vi "Move_Axis_tl.vi"(2 "GOTO":dbl step=1.0 format="%.5f", 3 "Mode":enum16{"Move", "Teach"}(ring), 4 "AXIS":T2 items=["Spare 0", "X", "Y", "Z", "THETA", "PHI", "Spare 6"]) -> (0 "ACTUAL POS.":dbl step=0.00125 format="%.5f", 1 "CURRENT POSITIONS":T1[](array[typedef])=[{"axis"="X", "mac position"=0.0}, {"axis"="Y", "mac position"=0.0}, {"axis"="Z", "mac position"=0.0}, {"axis"="PHI", "mac position"=0.0}, {"axis"="THETA", "mac position"=0.0}] {"mac position" format="%.5f"})   [LabVIEW 2010]
uses:
  TRAVERSE SUB-VIs/Custom Controls/Axis_Control_tl.ctl
  TRAVERSE SUB-VIs/Custom Controls/Axis_pos_cluster_tl.ctl
  TRAVERSE SUB-VIs/Functional VIs/Traverse_setup_tl.glob.vi
panel:
  in  "ADJUST PARAMETERS?":bool=TRUE
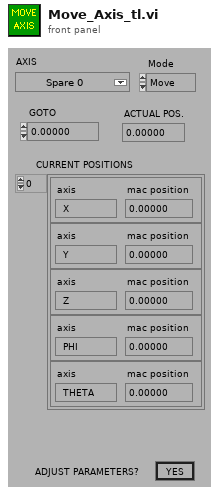
[diagram p1: front panel]
types:
  T1 = typedef "Axis_pos_cluster_tl.ctl" = cluster{"axis":string, "mac position":dbl}
  T2 = typedef "Axis_Control_tl.ctl" = u16
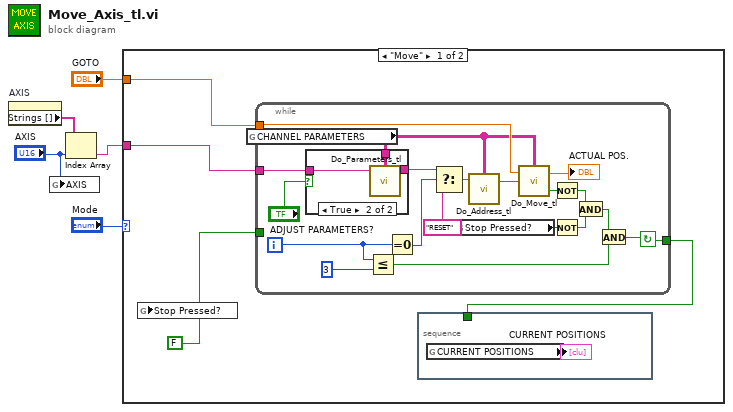
[diagram p0: block diagram]
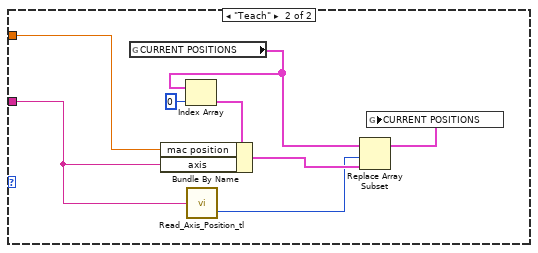
[diagram p3: hidden frame]
diagram:
  n1 = property on="AXIS" class="Ring (strict)"() -> ("Strings []"=w4:string[])  [unwired: 2 in, 2 out]
  n2 = global write "Traverse_setup_tl.glob.vi" "AXIS"("AXIS") -> ()
  n3 = Index Array(array=w4, index="AXIS") -> (element=w2:string)
  n4 = case shown="\"Move\"" "Mode" {
    tunnel: w2 -> [w8 w39]
    tunnel: "GOTO" -> [w6 w34]
    frame "Move" {
      w7 = FALSE
      n5 = global write "Traverse_setup_tl.glob.vi" "Stop Pressed?"(w7) -> ()
      n6 = while {
        tunnel: w7 -> [_]
        tunnel: [w15] -> w9
        tunnel: w8 -> [w21]
        tunnel: w6 -> [w26]
        i -> [w18]
        stop <- w15 continue-if-true
        n7 = global read "Traverse_setup_tl.glob.vi" "CHANNEL PARAMETERS"() -> (w19:string[][])
        n8 = case shown="True" "ADJUST PARAMETERS?" {
          tunnel: w19 -> [_ w32]
          tunnel: [w29 w31] -> w22
          tunnel: w21 -> [w29 w30]
          frame False {
          }
          frame True {
            n9 = call "Do_Parameters_tl.vi"("CHANNEL PARAMETERS"=w32, "Axis Name"=w30) -> ("Current Axis Name"=w31:string)  [unwired: 3 in]
          }
        }
        n10 = Less Or Equal?(x=w18, y=3) -> (x <= y?=w16:bool)
        n11 = Equal To 0?(x=w18) -> (x = 0?=w23:bool)
        n12 = Select(t=w22, s=w23, f="RESET") -> (s? t:f=w25:string)
        n13 = global read "Traverse_setup_tl.glob.vi" "Stop Pressed?"() -> (w13:bool)
        n14 = call "Do_Address_tl.vi"("CHANNEL PARAMETERS"=w19, "Axis Name"=w25) -> ("Current Axis Name"=w27:string)  [unwired: 3 in]
        n15 = call "Do_Move_tl.vi"("CHANNEL PARAMETERS"=w19, "Abs Pos REQD."=w26, "Axis Name"=w27) -> ("Move OK?"=w14:bool, "Abs Pos ACHVD."=→"ACTUAL POS.":dbl)  [unwired: 1 in]
        n16 = Not(x=w14) -> (.not. x?=w10:bool)
        n17 = Not(x=w13) -> (.not. x?=w12:bool)
        n18 = And(x=w10, y=w12) -> (x .and. y?=w11:bool)
        n19 = And(x=w11, y=w16) -> (x .and. y?=w15:bool)
      }
      n20 = stacked-sequence {
        tunnel: w9 -> [_]
        frame #0 {
          n21 = global read "Traverse_setup_tl.glob.vi" "CURRENT POSITIONS"() -> (→"CURRENT POSITIONS":T1[])
        }
      }
    }
    frame "Teach" {
      n22 = global read "Traverse_setup_tl.glob.vi" "CURRENT POSITIONS"() -> (w37:T1[])
      n23 = Index Array(array=w37, index=0) -> (element=w35:T1)
      n24 = Bundle By Name(cluster=w35, "mac position"=w34, "axis"=w39) -> (w41:T1)
      n25 = call "Read_Axis_Position_tl.vi"("Axis"=w39) -> ("Index"=w38:i32)  [unwired: 1 out]
      n26 = Replace Array Subset(array=w37, new element=w41, index=w38) -> (w40:T1[])
      n27 = global write "Traverse_setup_tl.glob.vi" "CURRENT POSITIONS"(w40) -> ()
    }
  }
